vi "mclb_hide_ants.vi"(8 "error in (no error)":errorcluster, 11 "mclb in":refnum<vi>) -> (0 "error out":errorcluster, 3 "mclb out":refnum<vi>)   [LabVIEW 2017, in "rywindow.lvclass"]
uses:
  rywindow.lvclass
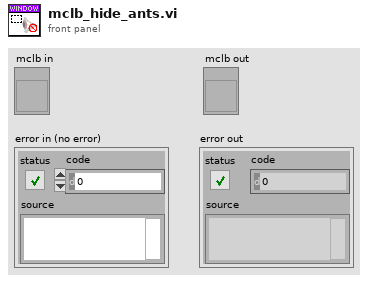
[diagram p1: front panel]
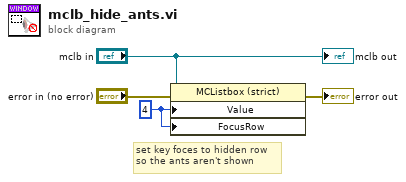
[diagram p0: block diagram]
diagram:
  w4 = 4 ("Value")
  # "set key foces to hidden row\nso the ants aren't shown"
  n1 = property class="MCListbox (strict)"(reference="mclb in", error in="error in (no error)", "Value"=w4, "FocusRow"=w4) -> (error out=→"error out":errorcluster)  [unwired: 1 out]
  "mclb out" <- "mclb in"
